vi "Enable Templating.vi"(7 "TemplateService (Basic)":refnum<class "TemplateService.lvclass">, 8 "error in (no error)":errorcluster, 9 "Default Index (index.html)":string="index.html", 10 "Root Folder":path, 11 "Server in":refnum<class "Server.lvclass">) -> (0 "error out":errorcluster, 3 "Server out":refnum<class "Server.lvclass">)   [LabVIEW 2020, in "HTTP Server.lvlib" / "Server.lvclass"]
uses:
  Server.lvclass
  TemplateService/TemplateService.lvclass
  C:/dev/lv20CE/relink/lv-http-server/HTTP Server/Service/Service.lvclass
  BasicTemplater/BasicTemplater.lvclass
  C:/dev/lv20CE/relink/lv-http-server/HTTP Server/TemplateService/TemplateService.lvclass
  TemplatedFileServe/TemplatedFileServe.lvclass
  C:/dev/lv20CE/relink/lv-http-server/HTTP Server/Handler/Handler.lvclass
  Add Connection Handler.vi
  Add Request Handler.vi
  Add Route Handler.vi
  Add Controller Handler.vi
  Add Controller.vi
  Add Response Handler.vi
  Add Complete Handler.vi
  Add Exception Handler.vi
  Connection Handler/Connection Handler.lvclass
  Request Handler/Request Handler.lvclass
  Route Handler/Route Handler.lvclass
  Controller Handler/Controller Handler.lvclass
  Controller/Controller.lvclass
  Response Handler/Response Handler.lvclass
  Complete Handler/Complete Handler.lvclass
  Exception Handler/Exception Handler.lvclass
  Handler/Handler.lvclass
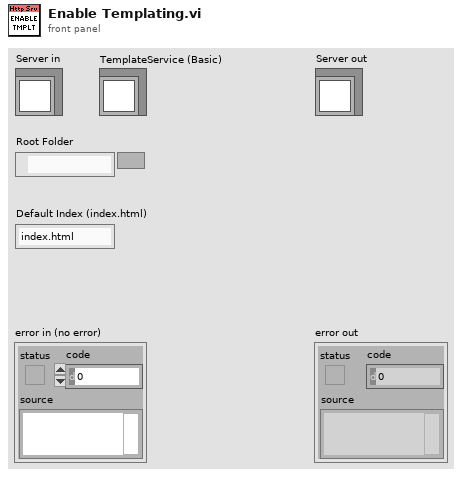
[diagram p1: front panel]
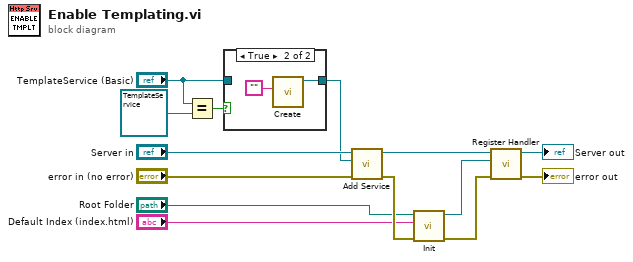
[diagram p0: block diagram]
diagram:
  n1 = Equal?(x="TemplateService (Basic)", y=refnum<class "TemplateService.lvclass"> refnum ("x")) -> (x = y?=w3:bool)
  n2 = case shown="True" w3 {
    tunnel: "TemplateService (Basic)" -> [w15 _]
    tunnel: [w15 w17] -> w1
    frame False {
    }
    frame True {
      n3 = call "Create.vi"("Default Namespace"="") -> ("BasicTemplater out"=w17:refnum<class "BasicTemplater.lvclass">)  [unwired: 9 in, 1 out]
    }
  }
  n4 = call "Add Service.vi"("error in (no error)"="error in (no error)", "Service"=w1, "Server in"="Server in") -> ("error out"=w14:errorcluster, "Server out"=w8:refnum<class "Server.lvclass">)  [unwired: 7 in]
  n5 = call "Init.vi"("error in (no error)"=w14, "Default Index File (index.html)"="Default Index (index.html)", "Public Root"="Root Folder") -> ("error out"=w5:errorcluster, "TemplatedFileServe out"=w6:refnum<class "TemplatedFileServe.lvclass">)  [unwired: 7 in]
  n6 = call "Register Handler.vi"("error in (no error)"=w5, "Handler"=w6, "Server in"=w8) -> ("error out"=→"error out":errorcluster, "Server out"=→"Server out":refnum<class "Server.lvclass">)  [unwired: 7 in]
